vi "FPGA Initial AD.vi"(8 "Error In":errorcluster, 11 "FPGA":T1) -> (0 "Error Out":errorcluster)   [LabVIEW 2017]
uses:
  WS_VCAP Driver 1_49/Source/WSVCAP Shell/Type Defs/WSVCAP SHL FPGA Enum.ctl
  WS_VCAP Driver 1_49/Source/WSVCAP Shell/Type Defs/WSVCAP SHL I2C DUT Mask Mode Enum.ctl
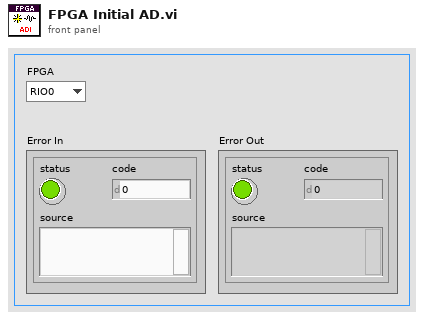
[diagram p1: front panel]
types:
  T1 = typedef "WSVCAP SHL FPGA Enum.ctl" = enum16{"RIO0", "RIO1"}
  T2 = typedef "WSVCAP SHL I2C DUT Mask Mode Enum.ctl" = enum16{"Custom", "All"}
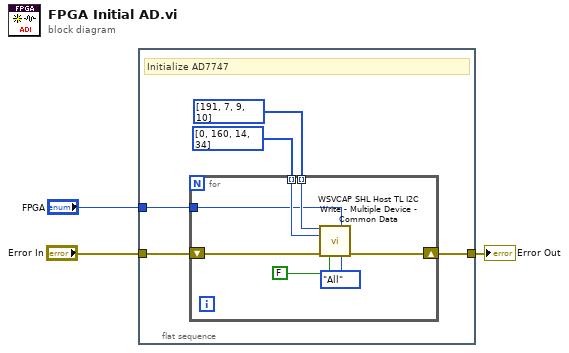
[diagram p0: block diagram]
diagram:
  n1 = flat-sequence {
    tunnel: "FPGA" -> [w6]
    tunnel: "Error In" -> [w5]
    tunnel: [w4] -> w1
    frame #0 {
      # "Initialize AD7747"
      n2 = for {
        tunnel: u8[] [191, 7, 9, 10] -> [w15] mode=indexing
        tunnel: u8[] [0, 160, 14, 34] -> [w14] mode=indexing
        tunnel: w6 -> [w13]
        shift-right: [w9] -> w4
        shift-left: w5 -> [w10]
        n3 = call "WSVCAP SHL Host TL I2C Write - Multiple Device - Common Data.vi"("Sub Address"=w15, "FPGA"=w13, "Data Out [U8]"=w14, "error in"=w10, "Log (T)"=FALSE, "DUT Mask Mode (All)"=WSVCAP_SHL_I2C_DUT_Mask_Mode_Enum."All") -> ("error out"=w9:errorcluster)  [unwired: 9 in]
      }
    }
  }
  "Error Out" <- w1
